vi "Main.vi"   [LabVIEW 2020]
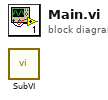
[diagram p0: block diagram]
diagram:
  n1 = call "SubVI.vi"() -> ()  [unwired: 12 in]
